vi "Test.vi"() -> ()   [LabVIEW 2015]
uses:
  Tagged Union.ctl
  <vilib>/Erdos Miller/LV-Tagged-Union/define-xnode/LV-Define-Tagged-Union.xnode
  <vilib>/Erdos Miller/LV-Tagged-Union/construct-xnode/LV-Construct-Tagged-Union.xnode
  <vilib>/Erdos Miller/LV-Tagged-Union/case-xnode/LV-Case-Tagged-Union.xnode
panel:
  in  "Tab Control":enum32{"String", "Number", "Bool Array"}(tab)
  in  "String":string
  in  "Number":dbl
  in  "Bool Array":bool[](array[boolean])
  out "Value":string
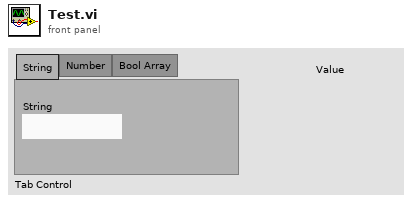
[diagram p1: front panel]
types:
  T1 = cluster{"Number":dbl, "Bool Array":bool[], "String":string}
  T2 = typedef "Tagged Union.ctl" = cluster{"\\type":enum32{"String", "Number", "Bool Array"}, "ÿýÿýÿýÿýÿý":variant}
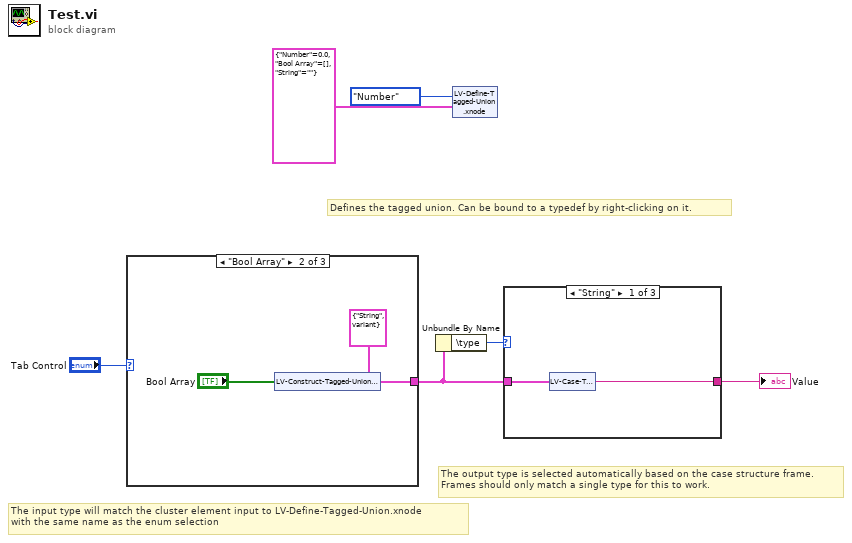
[diagram p0: block diagram]
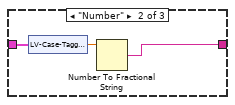
[diagram p2: hidden frame]
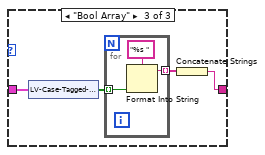
[diagram p3: hidden frame]
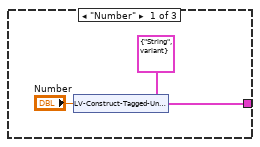
[diagram p4: hidden frame]
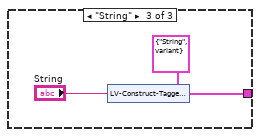
[diagram p5: hidden frame]
diagram:
  # "The output type is selected automatically based on the case structure frame.\nFrames should only match a single type for this to work."
  # "The input type will match the cluster element input to LV-Define-Tagged-Union.xnode\nwith the same name as the enum selection"
  # "Defines the tagged union. Can be bound to a typedef by right-clicking on it."
  n1 = case shown="\"Bool Array\"" "Tab Control" {
    tunnel: [w7 w15 w21] -> w5
    frame "Number" {
      n2 = xnode "LV-Construct-Tagged-Union.xnode"("Type"=T2 {"\\type"=enum."String", "ÿýÿýÿýÿýÿý"=variant} ("Cluster"), "in"="Number") -> ("Tagged Union out"=w7:T2)
    }
    frame "Bool Array" {
      n3 = xnode "LV-Construct-Tagged-Union.xnode"("Type"=T2 {"\\type"=enum."String", "ÿýÿýÿýÿýÿý"=variant} ("Cluster"), "in"="Bool Array") -> ("Tagged Union out"=w15:T2)
    }
    frame "String" {
      n4 = xnode "LV-Construct-Tagged-Union.xnode"("Type"=T2 {"\\type"=enum."String", "ÿýÿýÿýÿýÿý"=variant} ("Cluster"), "in"="String") -> ("Tagged Union out"=w21:T2)
    }
  }
  n5 = Unbundle By Name(w5) -> ("\\type"=w6:enum32{"String", "Number", "Bool Array"})
  n6 = xnode "LV-Define-Tagged-Union.xnode"("Enum"=enum32{"String", "Number", "Bool Array"}."Number" ("Tab Control"), "Types"=T1 {"Number"=0.0, "Bool Array"=[], "String"=""}) -> ()  [unwired: 1 out]
  n7 = case shown="\"String\"" w6 {
    tunnel: w5 -> [w29 w36 w44]
    tunnel: [w28 w34 w41] -> w2
    frame "String" {
      n8 = xnode "LV-Case-Tagged-Union.xnode"("Tagged Union in"=w29) -> ("Value out"=w28:string)
    }
    frame "Number" {
      n9 = xnode "LV-Case-Tagged-Union.xnode"("Tagged Union in"=w36) -> ("Value out"=w35:dbl)
      n10 = Number To Fractional String(number=w35) -> (F-format string=w34:string)  [unwired: 3 in]
    }
    frame "Bool Array" {
      n11 = xnode "LV-Case-Tagged-Union.xnode"("Tagged Union in"=w44) -> ("Value out"=w43:bool[])
      n12 = for {
        tunnel: w43 -> [w47] mode=indexing
        tunnel: [w45] -> w42 mode=indexing
        n13 = Format Into String(format string="%s ", w47) -> (resulting string=w45:string)  [unwired: 2 in, 1 out]
      }
      n14 = Concatenate Strings(w42) -> (w41:string)
    }
  }
  "Value" <- w2
